vi "Define Ramp Array Dialog.vi"(8 "error in (no error)":errorcluster) -> (0 "error out":errorcluster, 1 "OK?":bool caption="OK", 3 "Ramp":dbl[](array[numeric]))   [LabVIEW 2019]
doc: "Displays a standard dialog box that prompts users to enter information, such as a user name and password.\n--------------------\n\nThis Express VI is configured as follows:\n\nMessage to Display to the User:This is a test\nThe inputs are: \nNumber: Ramp Type\nNumber: Start\nNumber: End"
uses:
  <vilib>/Analysis/NI_AALBase.lvlib
panel:
  in  "Delta":dbl caption="Start" format="%#g"
  in  "Exclude End?":bool
  in  "Spacing":enum16{"Linear", "Logarithmic"}(ring)
  in  "Ramp Type":enum16{"Ramp by Sample", "Ramp by Delta"}(ring)
  in  "End":dbl format="%#g"
  in  "Start":dbl format="%#g"
  in  "# Samples":i32=1 caption="Ramp Type" min=1
  in  "Cancel":bool
  in  "OK":bool caption="OK2"
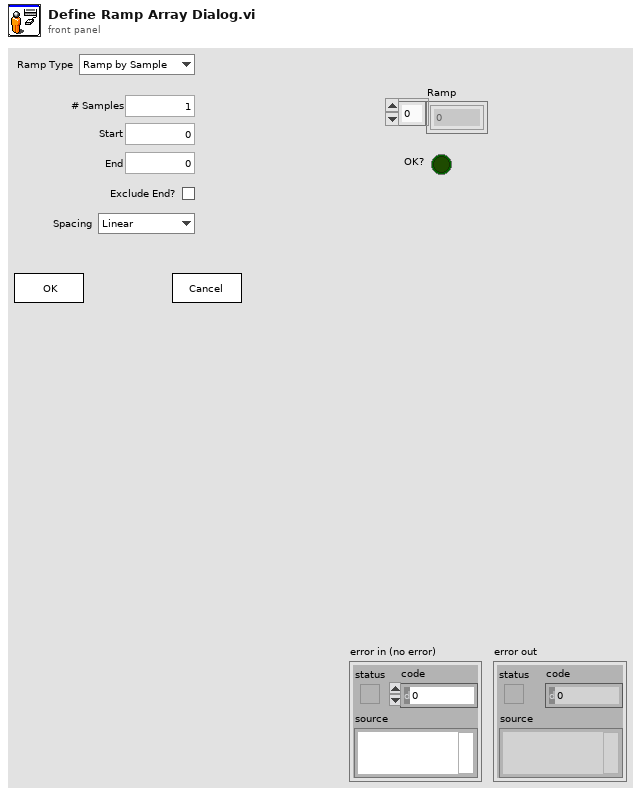
[diagram p1: front panel]
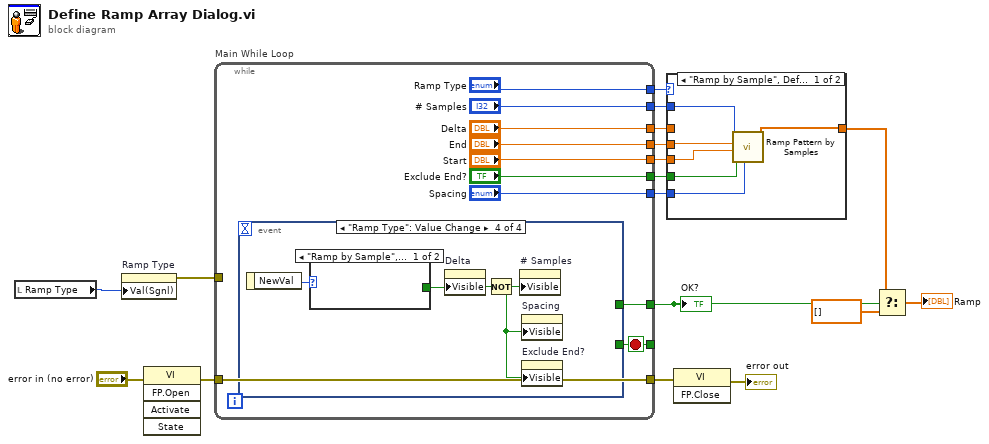
[diagram p0: block diagram]
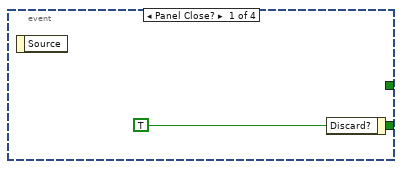
[diagram p2: hidden frame]
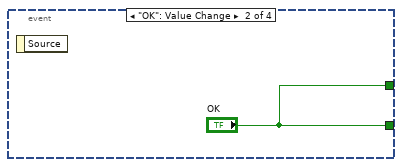
[diagram p3: hidden frame]
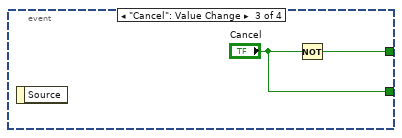
[diagram p4: hidden frame]
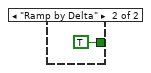
[diagram p5: hidden frame]
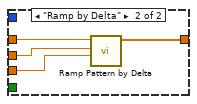
[diagram p6: hidden frame]
diagram:
  n1 = local read "Ramp Type"() -> (w2:enum16{"Ramp by Sample", "Ramp by Delta"})
  n2 = property on="Ramp Type" class="Enum (strict)"("Val(Sgnl)"=w2) -> (error out=w1:errorcluster)  [unwired: 2 in, 1 out]
  n3 = invoke class="VI" method="FP.Open"(error in="error in (no error)") -> (error out=w17:errorcluster)  [unwired: 4 in, 4 out]
  n4 = while "Main While Loop" {
    tunnel: w17 -> [w27]
    tunnel: [w27] -> w15
    tunnel: ["# Samples"] -> w9
    tunnel: [w25] -> _
    tunnel: ["Ramp Type"] -> w13
    tunnel: ["Delta"] -> w12
    tunnel: ["Start"] -> w11
    tunnel: ["End"] -> w10
    tunnel: ["Exclude End?"] -> w8
    tunnel: ["Spacing"] -> w7
    tunnel: [w18] -> w6
    tunnel: w1 -> [_]
    stop <- w25 stop-if-true
    n5 = event shown="[3] \"Ramp Type\": Value Change" {
      selector: _ -> [_ _ _ _]
      dyn-events: _ -> [_ _ _ _]
      timeout: _ -> [_ _ _ _]
      tunnel: [w28 "OK" "Cancel" _] -> w25
      tunnel: [_ "OK" w30 _] -> w18
      event Panel Close? {
        w28 = TRUE ("Discard?")
        n6 = event-data() -> ()  [unwired: 1 in, 1 out]
        n7 = event-data("Discard?"=w28) -> ()  [unwired: 1 in, 1 out]
      }
      event "OK": Value Change {
        n8 = event-data() -> ()  [unwired: 1 in, 1 out]
      }
      event "Cancel": Value Change {
        n9 = event-data() -> ()  [unwired: 1 in, 1 out]
        n10 = Not(x="Cancel") -> (.not. x?=w30:bool)
      }
      event "Ramp Type": Value Change {
        n11 = event-data() -> ("NewVal"=w34:enum16{"Ramp by Sample", "Ramp by Delta"})  [unwired: 1 in]
        n12 = case shown="\"Ramp by Sample\", Default" w34 {
          tunnel: [_ TRUE ("Visible")] -> w33
          frame "Ramp by Sample", Default {
          }
          frame "Ramp by Delta" {
          }
        }
        n13 = property on="Delta" class="DigNum (strict)"("Visible"=w33) -> ()  [unwired: 2 in, 2 out]
        n14 = Not(x=w33) -> (.not. x?=w32:bool)
        n15 = property on="# Samples" class="DigNum (strict)"("Visible"=w32) -> ()  [unwired: 2 in, 2 out]
        n16 = property on="Spacing" class="Enum (strict)"("Visible"=w32) -> ()  [unwired: 2 in, 2 out]
        n17 = property on="Exclude End?" class="Bool (strict)"("Visible"=w32) -> ()  [unwired: 2 in, 2 out]
      }
    }
  }
  "OK?" <- w6
  n18 = case shown="\"Ramp by Sample\", Default" w13 {
    tunnel: w12 -> [_ w45]
    tunnel: w11 -> [w39 w44]
    tunnel: w10 -> [w40 w43]
    tunnel: [w36 w42] -> w5
    tunnel: w9 -> [w41 _]
    tunnel: w8 -> [w38 _]
    tunnel: w7 -> [w37 _]
    frame "Ramp by Sample", Default {
      n19 = call <vilib>:"Ramp Pattern by Samples.vi"("type"=w37, "exclude end?"=w38, "start"=w39, "end"=w40, "samples"=w41) -> ("Ramp Pattern"=w36:dbl[])  [unwired: 5 in, 1 out]
    }
    frame "Ramp by Delta" {
      n20 = call <vilib>:"Ramp Pattern by Delta.vi"("start"=w44, "end"=w43, "delta"=w45) -> ("Ramp Pattern"=w42:dbl[])  [unwired: 6 in, 2 out]
    }
  }
  n21 = invoke class="VI" method="FP.Close"(error in=w15) -> (error out=→"error out":errorcluster)  [unwired: 2 in, 2 out]
  n22 = Select(t=w5, s=w6, f=dbl[] []) -> (s? t:f=→"Ramp":dbl[])
